vi "WPI_CameraWait for Raw Image String.vi"(8 "error in (no error)":errorcluster, 10 "Timeout in ms (-1)":i32=-1, 11 "CameraDevRef":T1) -> (0 "error out":errorcluster, 2 "String":string, 3 "CameraDevRef Out":T1)   [LabVIEW 2017]
doc: "This software is licensed. Open the labview\\readme\\WPI Robotics Library Open Source License.txt file for more information."
uses:
  <vilib>/Rock Robotics/WPI/Camera/WPI_CameraDevRef.ctl
  <vilib>/Rock Robotics/WPI/Camera/WPI_CameraSettings Operations.ctl
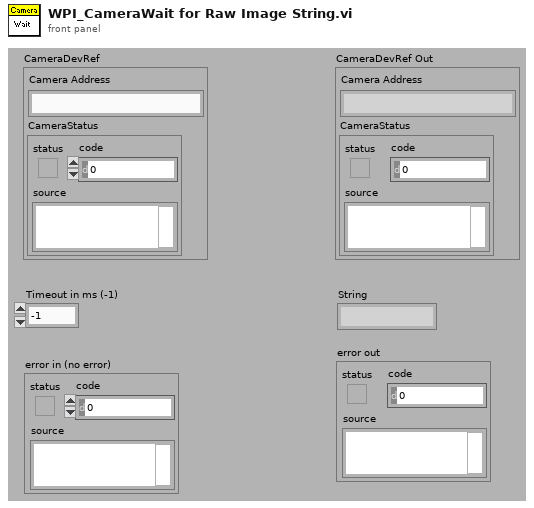
[diagram p1: front panel]
types:
  T1 = typedef "WPI_CameraDevRef.ctl" = cluster{"Camera Address":string, "CameraStatus":errorcluster}
  T2 = typedef "WPI_CameraSettings Operations.ctl" = enum16{"Udate FPS", "Update Compression", "Update Size", "Update White Balance", "Update Brightness", "Update Sharpness", "Update Exposure", "Update Exposure Value", "Update Color Level", "Update Exp Priority", "Update Color Enable", "Update JPG", "Update MJPG", "Read and Clear", "Read", "Init"}
  T3 = typedef "WPI_CameraSettings Control.ctl" = cluster{"FPS":i32, "Compression":i32, "Size":i32, "White Balance":i32, "Brightness":i32, "Sharpness":i32, "Exposure":i32, "Color Level":i32, "Exposure Priority":i32, "Color Enable":i32, "JPG Loop":i32, "MJPG Loop":i32, "Exposure Value":i32}
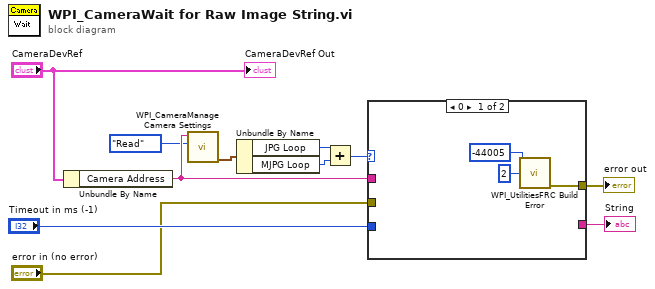
[diagram p0: block diagram]
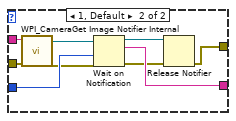
[diagram p2: hidden frame]
diagram:
  n1 = Unbundle By Name("CameraDevRef") -> ("Camera Address"=w6:string)
  n2 = call <vilib>:"WPI_CameraManage Camera Settings.vi"("Operation"=WPI_CameraSettings_Operations."Read", "Camera IP"=w6) -> ("Values"=w4:T3)  [unwired: 8 in, 1 out]
  n3 = Unbundle By Name(w4) -> ("JPG Loop"=w3:i32, "MJPG Loop"=w2:i32)
  n4 = Add(x=w3, y=w2) -> (x+y=w1:i32)
  n5 = case shown="0" w1 {
    tunnel: [_ w23] -> w11
    tunnel: "Timeout in ms (-1)" -> [_ w22]
    tunnel: [w12 w19] -> w9
    tunnel: w6 -> [_ w16]
    tunnel: "error in (no error)" -> [_ w15]
    frame 0 {
      n6 = call <vilib>:"WPI_UtilitiesFRC Build Error.vi"("error code"=-44005 ("code"), "chain levels to remove (1)"=2) -> ("error out"=w12:errorcluster)  [unwired: 3 in, 10 out]
    }
    frame 1, Default {
      n7 = call <vilib>:"WPI_CameraGet Image Notifier Internal.vi"("error in (no error)"=w15, "Camera Address"=w16) -> ("error out"=w18:errorcluster, "Image Notifier"=w17:refnum<notifier>)  [unwired: 8 out]
      n8 = Wait on Notification(notifier=w17, timeout in ms (-1)=w22, error in (no error)=w18) -> (notifier out=w21:refnum<notifier>, notification=w23:string, error out=w20:errorcluster)  [unwired: 2 out]
      n9 = Release Notifier(notifier=w21, error in (no error)=w20) -> (error out=w19:errorcluster)  [unwired: 3 out]
    }
  }
  "error out" <- w9
  "String" <- w11
  "CameraDevRef Out" <- "CameraDevRef"
